vi "完全平方数.vi"(11 "范围":i32=100) -> (3 "平方数":i32[](array[numeric]))   [LabVIEW 2012]
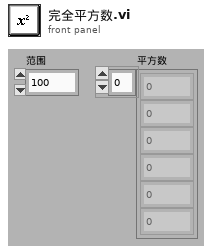
[diagram p1: front panel]
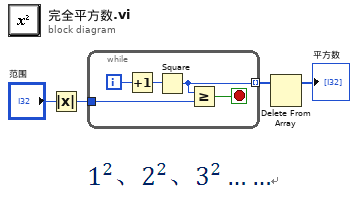
[diagram p0: block diagram]
diagram:
  n1 = Absolute Value(x="范围") -> (abs(x)=w2:i32)
  n2 = while {
    tunnel: w2 -> [w9]
    tunnel: [w5] -> w4 mode=indexing
    i -> [w7]
    stop <- w8 stop-if-true
    n3 = Increment(x=w7) -> (x+1=w6:i32)
    n4 = Square(x=w6) -> (x^2=w5:i32)
    n5 = Greater Or Equal?(x=w5, y=w9) -> (x >= y?=w8:bool)
  }
  n6 = Delete From Array(array=w4) -> (array with subset deleted=→"平方数":i32[])  [unwired: 2 in, 1 out]
